vi "Read MenuRef.vi"(8 "error in (no error)":errorcluster, 11 "ShortcutMenuActivationMsg in":refnum<class "ShortcutMenuActivationMsg.lvclass">) -> (0 "error out":errorcluster, 2 "MenuRef":refnum<k9>, 3 "ShortcutMenuActivationMsg out":refnum<class "ShortcutMenuActivationMsg.lvclass">)   [LabVIEW 2020, in "ActorEvents.lvlib" / "ShortcutMenuActivationMsg.lvclass"]
uses:
  <vilib>/gpm_packages/@cs/mva-viewable/Source/ActorEvents/IEventAggregator Messages/ShortcutMenuActivationMsg/ShortcutMenuActivationMsg.lvclass
  <vilib>/gpm_packages/@cs/mva-viewable/Source/ActorEvents/IEventAggregator Messages/ShortcutMenuActivationMsg/ShortcutMenuActivationMsg.lvclass/ShortcutMenuActivationMsg.ctl
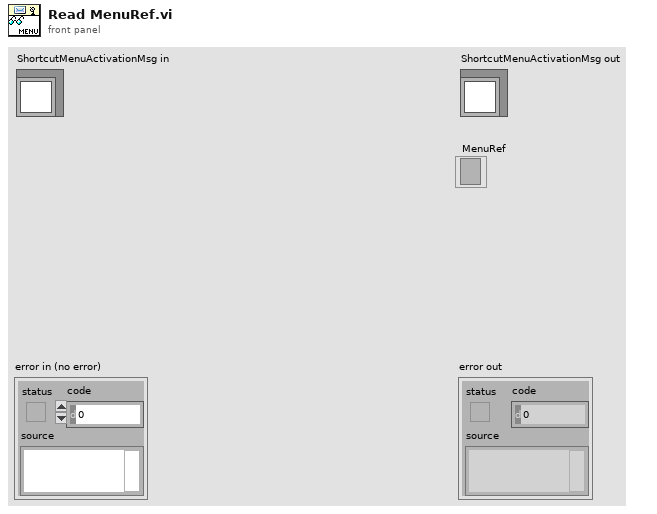
[diagram p1: front panel]
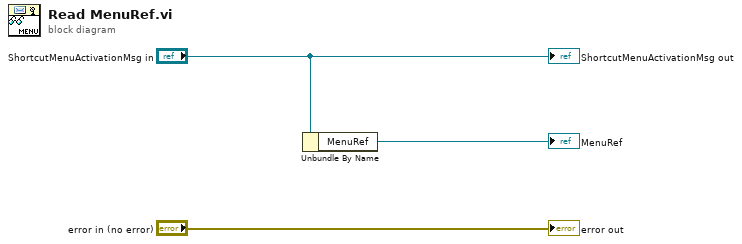
[diagram p0: block diagram]
diagram:
  n1 = Unbundle By Name("ShortcutMenuActivationMsg in") -> ("MenuRef"=→"MenuRef":refnum<k9>)
  "error out" <- "error in (no error)"
  "ShortcutMenuActivationMsg out" <- "ShortcutMenuActivationMsg in"
